vi "calculate_v.vi"(0 "Z0":dbl, 1 "mic4灵敏度Sen(V/Pa)":dbl, 2 "S_factor":cdb, 5 "L[mm]":dbl, 7 "Rate":i32, 9 "mic4":dbl[](array[numeric]), 11 "dia_tube(m)":dbl, 12 "c0":dbl) -> (4 "V":cdb[](array[numeric]), 8 "f":dbl[](array[numeric]))   [LabVIEW 2018]
uses:
  <vilib>/Analysis/2dsp.llb/Real FFT.vi
  <vilib>/Analysis/NI_AALPro.lvlib
panel:
  out "IM":cluster{"X":dbl, "Y":dbl}[](graph)
  out "RE":cluster{"X":dbl, "Y":dbl}[](graph)
  out "波形图表":waveform(dbl)(graph)
  out "XY图 2":cluster{"X":dbl, "Y":dbl}[](graph)
  out "XY图":cluster{"X":dbl, "Y":dbl}[](graph)
  in  "滑动活塞距离L(mm)":dbl
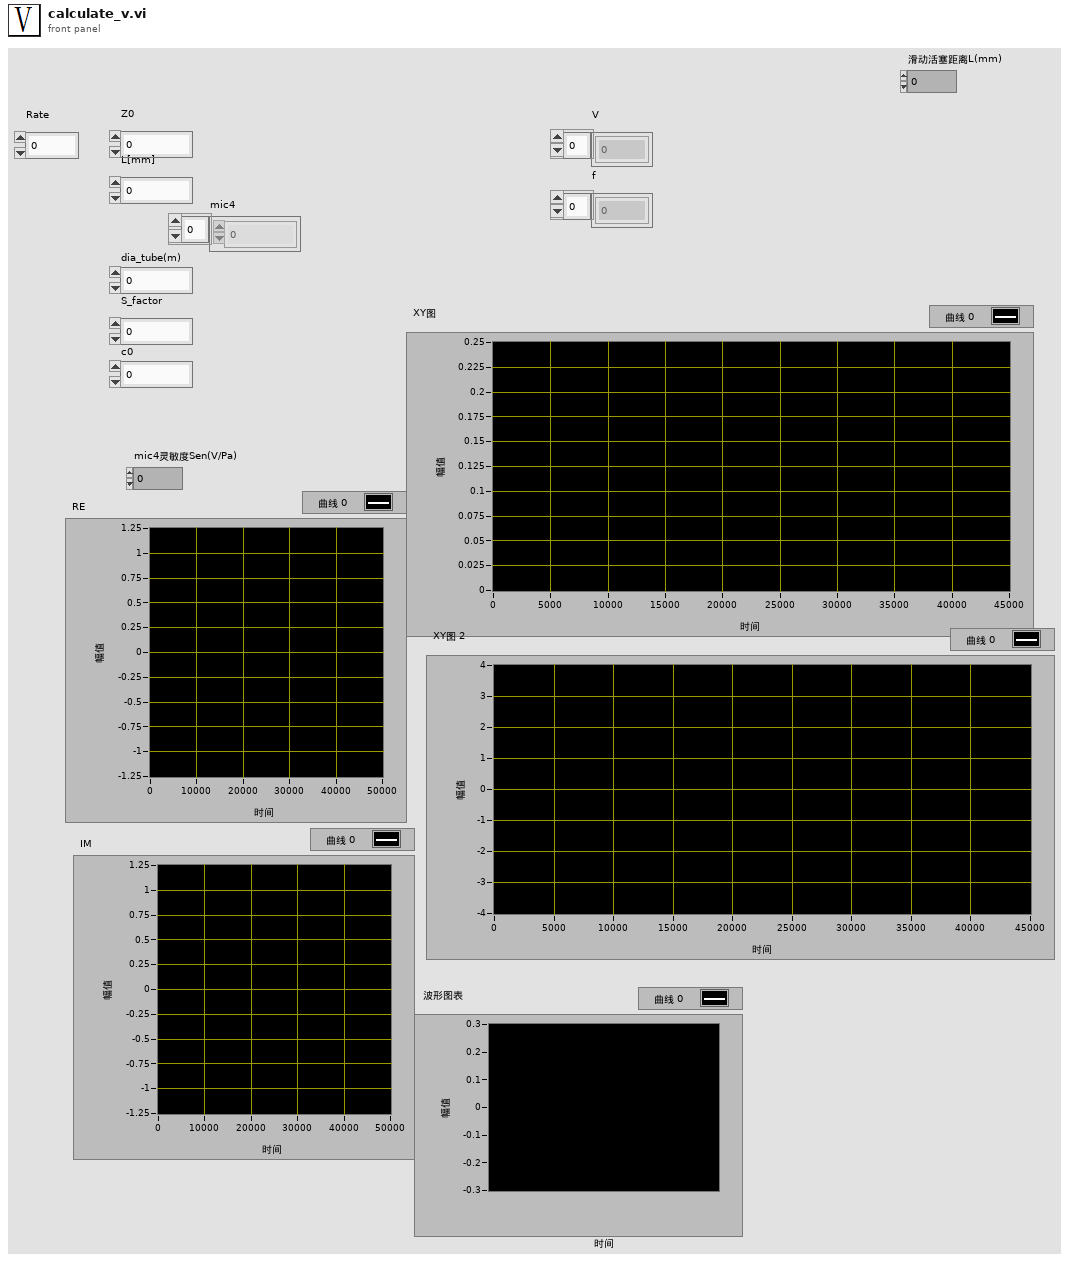
[diagram p1: front panel]
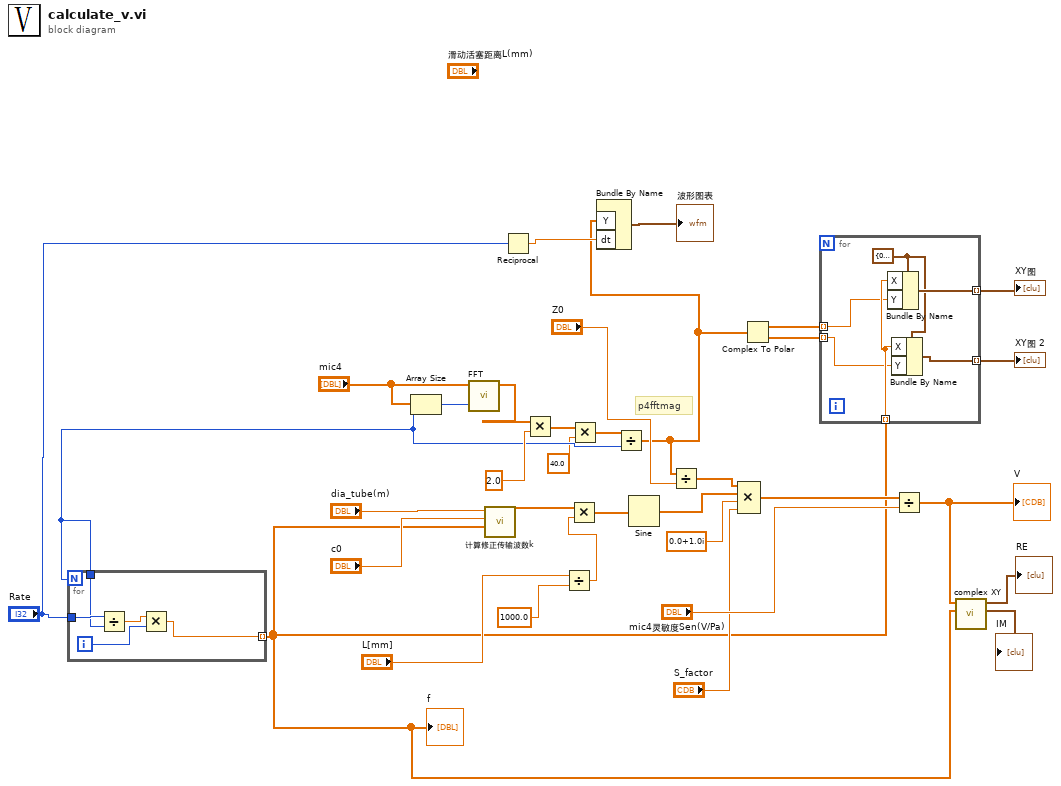
[diagram p0: block diagram]
diagram:
  # "p4fftmag"
  n1 = Array Size(array="mic4") -> (size(s)=w14:i32)
  n2 = for {
    N: w14 -> [_]
    tunnel: "Rate" -> [w38]
    tunnel: [w34] -> w6 mode=indexing
    tunnel: w14 -> [w37]
    i -> [w36]
    n3 = Divide(x=w38, y=w37) -> (x/y=w35:dbl)
    n4 = Multiply(x=w35, y=w36) -> (x*y=w34:dbl)
  }
  "f" <- w6
  n5 = call-poly <vilib>:"FFT.vi"("FFT size"=w14, "X"="mic4") -> ("FFT {X}"=w17:cdb[])  [unwired: 8 in, 1 out]
  n6 = call "计算修正传输波数k.vi"("f"=w6, "c0"="c0", "dia_tube(m)"="dia_tube(m)") -> ("k"=w8:cdb[])  [unwired: 8 in]
  n7 = Reciprocal(x="Rate") -> (1/x=w10:dbl)
  n8 = Multiply(x=w17, y=2.0) -> (x*y=w2:cdb[])
  n9 = Divide(x="L[mm]", y=1000.0) -> (x/y=w33:dbl)
  n10 = Multiply(x=w8, y=w33) -> (x*y=w28:cdb[])
  n11 = Multiply(x=w2, y=40.0) -> (x*y=w3:cdb[])
  n12 = Divide(x=w3, y=w14) -> (x/y=w9:cdb[])
  n13 = Bundle By Name("Y"=w9, "dt"=w10) -> (→"波形图表":waveform(cdb))  [unwired: 1 in]
  n14 = Sine(x=w28) -> (sin(x)=w29:cdb[])
  n15 = Divide(x=w9, y="Z0") -> (x/y=w26:cdb[])
  n16 = Compound Arithmetic op=MULTIPLY(w26, w29, cdb 0.0+1.0i, "S_factor") -> (w30:cdb[])
  n17 = Complex To Polar(r * e^(i*theta)=w9) -> (r=w16:dbl[], theta=w15:dbl[])
  n18 = for {
    tunnel: [w44] -> w19 mode=indexing
    tunnel: [w42] -> w18 mode=indexing
    tunnel: w6 -> [w41] mode=indexing
    tunnel: w16 -> [w40] mode=indexing
    tunnel: w15 -> [w39] mode=indexing
    w43 = cluster{"X":dbl, "Y":dbl} {"X"=0.0, "Y"=0.0}
    n19 = Bundle By Name(cluster=w43, "X"=w41, "Y"=w40) -> (w44:cluster{"X":dbl, "Y":dbl})
    n20 = Bundle By Name(cluster=w43, "X"=w41, "Y"=w39) -> (w42:cluster{"X":dbl, "Y":dbl})
  }
  "XY图" <- w19
  "XY图 2" <- w18
  n21 = Divide(x=w30, y="mic4灵敏度Sen(V/Pa)") -> (x/y=w7:cdb[])
  "V" <- w7
  n22 = call "complex XY.vi"("f"=w6, "数组"=w7) -> ("IM"=→"IM":cluster{"X":dbl, "Y":dbl}[], "RE"=→"RE":cluster{"X":dbl, "Y":dbl}[])  [unwired: 8 in]
